vi "Polish BD Constant.vi"(10 "BD Const":refnum<vi>, 11 "Number Writer in":refnum<class "Number Writer.lvclass">) -> (3 "Number Writer out":refnum<class "Number Writer.lvclass">)   [LabVIEW 2013, in "Number Writer.lvclass"]
uses:
  Number Writer.lvclass
  Number Writer.lvclass/Number Writer.ctl
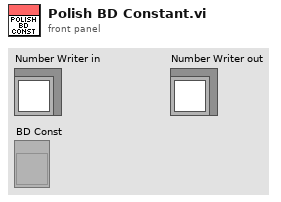
[diagram p1: front panel]
types:
  T1 = typedef "Number Writer.lvclass/Numeric Type.ctl" = enum16{"I8", "I16", "I32", "I64", "U8", "U16", "U32", "U64", "SGL", "DBL", "PTR INT", "PTR UINT"}
  T2 = typedef "LVNumericRepresentation.ctl" = enum32{"Extended Precision", "Double Precision", "Single Precision", "Long", "Word", "Byte", "Unsigned Long", "Unsigned Word", "Unsigned Byte", "Complex Extended", "Complex Double", "Complex Single", "Quad", "Unsigned Quad", "Fixed-Point"}
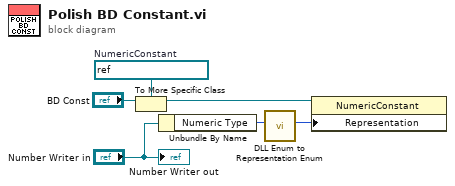
[diagram p0: block diagram]
diagram:
  w6 = refnum<vi> refnum  # NumericConstant
  n1 = To More Specific Class(target class=w6, reference="BD Const") -> (specific class reference=w2:refnum<vi>)  [unwired: 1 in, 1 out]
  n2 = Unbundle By Name("Number Writer in") -> ("Numeric Type"=w3:T1)
  n3 = call "DLL Enum to Representation Enum.vi"("Numeric Type"=w3) -> ("Representation"=w1:T2)  [unwired: 10 in]
  n4 = property class="NumericConstant"(reference=w2, "Representation"=w1) -> ()  [unwired: 1 in, 2 out]
  "Number Writer out" <- "Number Writer in"
